vi "ModeMgr.Save Mode Config.vi"(8 "Use DIalog":bool, 9 "Path":path, 10 "Modes":T1[](array[typedef]) {"Color" items=["Red", "Yellow", "Orange", "Green", "SkyBlue", "Blue", "Purple", "Pink", "Grey"]}, 11 "Default Mode":string="Production") -> ()   [LabVIEW 2018]
uses:
  ModeMgr.Mode Settings_Config View.ctl
  ModeMgr.Mode Settings.ctl
  ModeMgr.ModeConfig.ctl
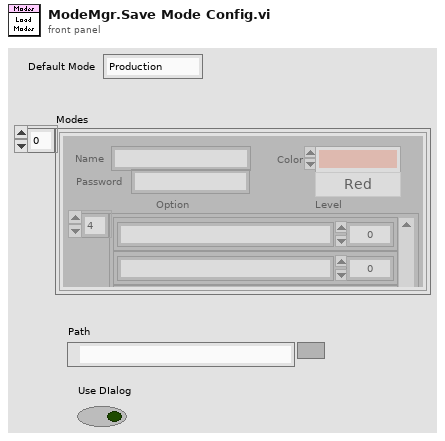
[diagram p1: front panel]
types:
  T1 = typedef "ModeMgr.Mode Settings_Config View.ctl" = cluster{"Name":string, "Color":u16, "Options":T2[], "Password":string}
  T2 = typedef "ModeMgr.Mode Settings.ctl" = cluster{"Option":string, "Level":i32}
  T3 = typedef "ModeMgr.ModeConfig.ctl" = cluster{"Name":string, "Color":string, "Settings":T2[], "Password":string}
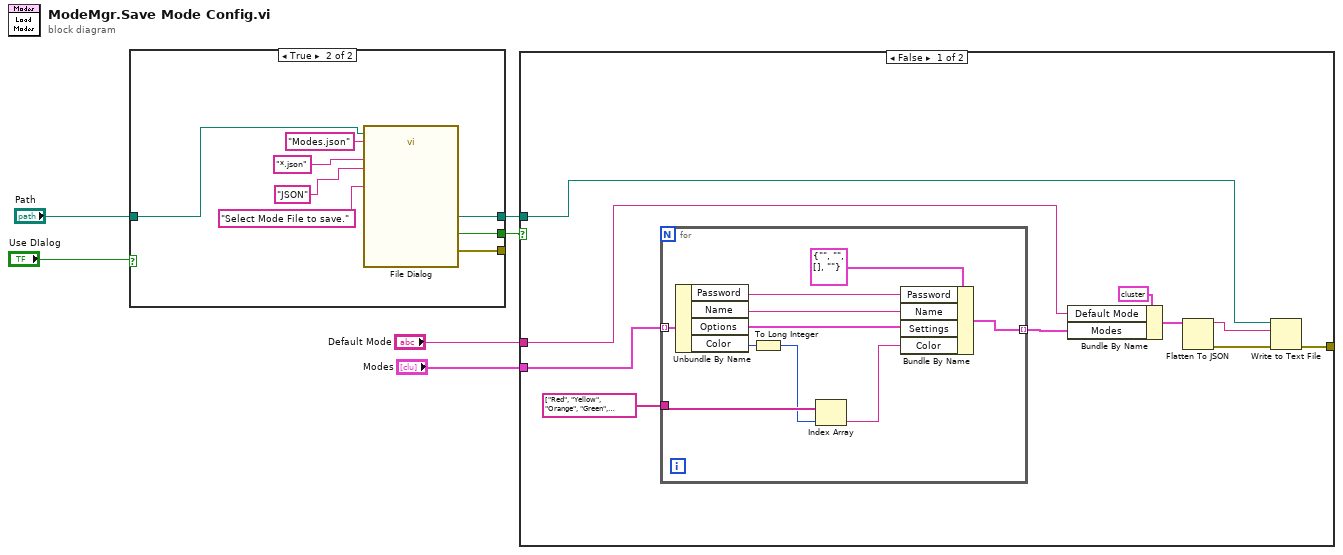
[diagram p0: block diagram]
diagram:
  n1 = case shown="True" "Use DIalog" {
    tunnel: [w7 w11] -> w6
    tunnel: "Path" -> [w7 w10]
    tunnel: [_ w9] -> w4
    tunnel: [_ w8] -> _
    frame False {
    }
    frame True {
      n2 = call "File Dialog"("start path"=w10, "prompt"="Select Mode File to save." ("prompt (Choose or enter file path)"), "default name"="Modes.json", "pattern (all files)"="*.json", "pattern label"="JSON" ("pattern (all files)")) -> ("selected path"=w11:path, "cancelled"=w9:bool, "error out"=w8:errorcluster)  [unwired: 7 in, 1 out]
    }
  }
  n3 = case shown="False" w4 {
    tunnel: w6 -> [w16 _]
    tunnel: "Default Mode" -> [w19 _]
    tunnel: "Modes" -> [w18 _]
    tunnel: [w17 _] -> _
    frame False {
      n4 = for {
        tunnel: w18 -> [w35] mode=indexing
        tunnel: string[] ["Red", "Yellow", "Orange", "Green", "SkyBlue", "Blue", "Purple", "Pink", "Grey"] ("Names") -> [w30]
        tunnel: [w32] -> w22 mode=indexing
        n5 = Unbundle By Name(w35) -> ("Password"=w26:string, "Name"=w34:string, "Options"=w33:T2[], "Color"=w29:u16)
        n6 = To Long Integer(number=w29) -> (32bit integer=w28:i32)
        n7 = Index Array(array=w30, index=w28) -> (element=w27:string)
        n8 = Bundle By Name(cluster=T3 {"Name"="", "Color"="", "Settings"=[], "Password"=""} ("Config"), "Password"=w26, "Name"=w34, "Settings"=w33, "Color"=w27) -> (w32:T3)
      }
      n9 = Bundle By Name(cluster=cluster{"Default Mode":string, "Modes":T3[]} {"Default Mode"="Production", "Modes"=[{"Name"="Production", "Color"="Green", "Settings"=[{"Option"="PreTest_Validate_SN", "Level"=1}, {"Option"="PostTest_ReportResult", "Level"=1}, {"Option"="OptTo_NotSaveResults", "Level"=0}, {"Option"="OptTo_NotStopOnFail", "Level"=0}, {"Option"="OptTo_SetConfig", "Level"=0}, {"Option"="OptTo_UpdateEquipmentList", "Level"=0}, {"Option"="OptTo_AccessManualStaControl", "Level"=0}], "Password"=""}, {"Name"="Technician", "Color"="Yellow", "Settings"=[{"Option"="PreTest_Validate_SN", "Level"=0}, {"Option"="PostTest_ReportResult", "Level"=0}, {"Option"="OptTo_NotSaveResults", "Level"=1}, {"Option"="OptTo_NotStopOnFail", "Level"=1}, {"Option"="OptTo_SetConfig", "Level"=0}, {"Option"="OptTo_UpdateEquipmentList", "Level"=0}, {"Option"="OptTo_AccessManualStaControl", "Level"=0}], "Password"=""}, {"Name"="Engineering", "Color"="SkyBlue", "Settings"=[{"Option"="PreTest_Validate_SN", "Level"=0}, {"Option"="PostTest_ReportResult", "Level"=0}, {"Option"="OptTo_NotSaveResults", "Level"=1}, {"Option"="OptTo_NotStopOnFail", "Level"=1}, {"Option"="OptTo_SetConfig", "Level"=1}, {"Option"="OptTo_UpdateEquipmentList", "Level"=1}, {"Option"="OptTo_AccessManualStaControl", "Level"=1}], "Password"=""}, {"Name"="Production", "Color"="Green", "Settings"=[], "Password"=""}, {"Name"="Technician", "Color"="Yellow", "Settings"=[], "Password"=""}, {"Name"="Engineering", "Color"="Blue", "Settings"=[], "Password"=""}]} ("Mode Config"), "Default Mode"=w19, "Modes"=w22) -> (w23:cluster{"Default Mode":string, "Modes":T3[]})
      n10 = Flatten To JSON(anything=w23) -> (JSON string=w24:string, 11:w25:errorcluster)  [unwired: 2 in]
      n11 = Write to Text File(file (use dialog)=w16, text=w24, error in=w25) -> (error out=w17:errorcluster)  [unwired: 1 in, 2 out]
    }
    frame True {
      # "Canceled"
    }
  }
